vi "Close VI FP.vi"(8 "error in":errorcluster, 9 "close all VI panels? (F)":bool, 10 "VI name (\"\")":string, 11 "state in":T1) -> (0 "error out":errorcluster, 3 "state out":T1)   [LabVIEW 2010, in "NI_SE_Config Front Panel Layout.lvlib"]
uses:
  NI_SE_Config Front Panel Layout.lvlib
  State.ctl
  VI Info.ctl
  VI Panel Layout/VI Panel Layout.lvclass
  Get VI Info Index by Name.vi
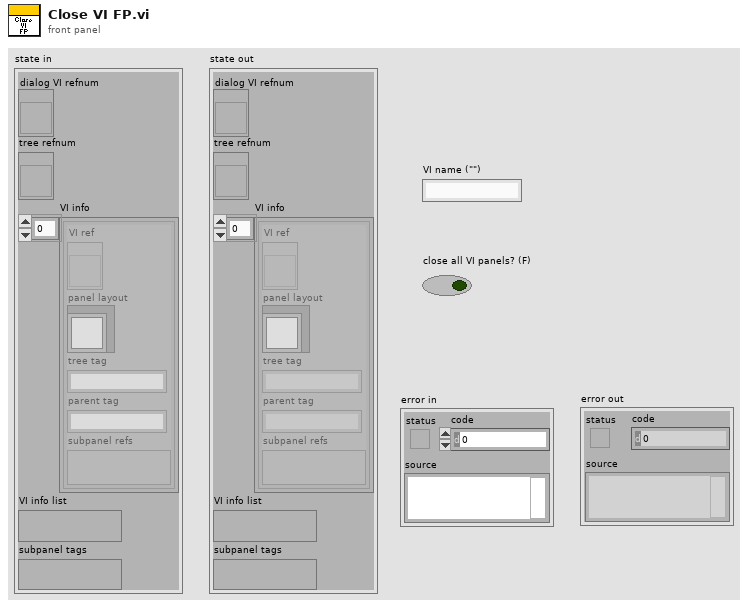
[diagram p1: front panel]
types:
  T1 = typedef "NI_SE_Config Front Panel Layout.lvlib/State.ctl" = cluster{"dialog VI refnum":refnum<vi>, "tree refnum":refnum<vi>, "VI info":T2[], "VI info list":variant, "subpanel tags":variant}
  T2 = typedef "NI_SE_Config Front Panel Layout.lvlib/VI Info.ctl" = cluster{"VI ref":refnum<vi>, "panel layout":refnum<class "VI Panel Layout.lvclass">, "tree tag":string, "parent tag":string, "subpanel refs":variant}
  T3 = enum32{"Invalid", "Standard", "Closed", "Hidden", "Minimized", "Maximized"}
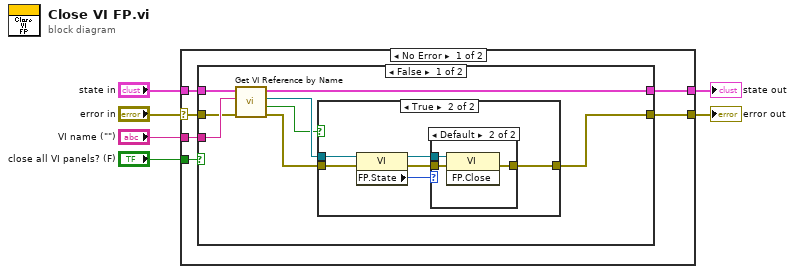
[diagram p0: block diagram]
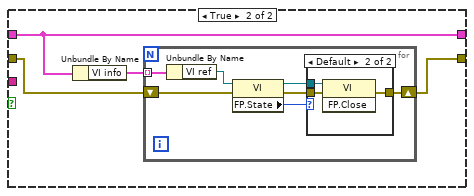
[diagram p4: hidden frame]
diagram:
  n1 = case shown="No Error" "error in" {
    selector: "error in" -> [w11 w47]
    tunnel: "state in" -> [w12 w48]
    tunnel: [w8 w48] -> w4
    tunnel: [w9 w47] -> w3
    tunnel: "VI name (\"\")" -> [w10 _]
    tunnel: "close all VI panels? (F)" -> [w7 _]
    frame No Error {
      n2 = case shown="False" w7 {
        tunnel: w12 -> [w19 w34]
        tunnel: w11 -> [w13 w33]
        tunnel: w10 -> [w18 _]
        tunnel: [w20 w32] -> w9
        tunnel: [w14 w34] -> w8
        frame False {
          n3 = call "Get VI Reference by Name.vi"("error in"=w13, "VI name"=w18, "state in"=w19) -> ("error out"=w15:errorcluster, "found?"=w16:bool, "VI ref"=w17:refnum<vi>, "state out"=w14:T1)  [unwired: 5 in]
          n4 = case shown="True" w16 {
            tunnel: w15 -> [w21 w24]
            tunnel: [w21 w23] -> w20
            tunnel: w17 -> [_ w22]
            frame False {
            }
            frame True {
              n5 = property class="VI"(reference=w22, error in=w24) -> (reference out=w27:refnum<vi>, error out=w25:errorcluster, "FP.State"=w26:T3)
              n6 = case shown="Default" w26 {
                tunnel: w25 -> [w28 w31]
                tunnel: [w28 w30] -> w23
                tunnel: w27 -> [_ w29]
                frame "Closed" {
                }
                frame Default {
                  n7 = invoke class="VI" method="FP.Close"(reference=w29, error in=w31) -> (error out=w30:errorcluster)  [unwired: 1 in, 2 out]
                }
              }
            }
          }
        }
        frame True {
          n8 = Unbundle By Name(w34) -> ("VI info"=w35:T2[])
          n9 = for {
            tunnel: w35 -> [w42] mode=indexing
            shift-right: [w41] -> w32
            shift-left: w33 -> [w37]
            n10 = Unbundle By Name(w42) -> ("VI ref"=w40:refnum<vi>)
            n11 = property class="VI"(reference=w40, error in=w37) -> (reference out=w39:refnum<vi>, error out=w36:errorcluster, "FP.State"=w38:T3)
            n12 = case shown="Default" w38 {
              tunnel: w36 -> [w43 w46]
              tunnel: [w43 w45] -> w41
              tunnel: w39 -> [_ w44]
              frame "Closed" {
              }
              frame Default {
                n13 = invoke class="VI" method="FP.Close"(reference=w44, error in=w46) -> (error out=w45:errorcluster)  [unwired: 1 in, 2 out]
              }
            }
          }
        }
      }
    }
    frame Error {
    }
  }
  "state out" <- w4
  "error out" <- w3
